vi "SaveVI.vi"(0 "VI in":refnum<vi>, 5 "Project Path":path, 7 "Folder name":string, 9 "VI name":string, 11 "error in (no error)":errorcluster) -> (4 "VI out":refnum<vi>, 15 "error out":errorcluster)   [LabVIEW 2016, in "ScriptSubVIs.lvlib"]
doc: "Creates and saves the New VI in a given name"
uses:
  ScriptSubVIs.lvlib
  <vilib>/SLL Toolkit/SLL File IO/SLL File IO.lvlib
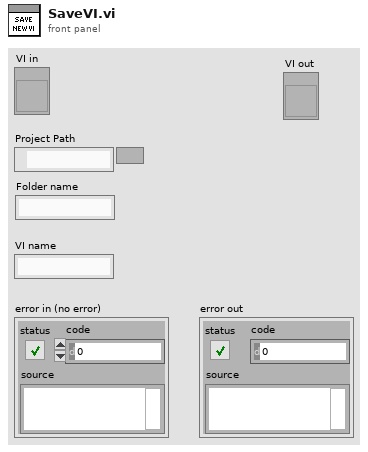
[diagram p1: front panel]
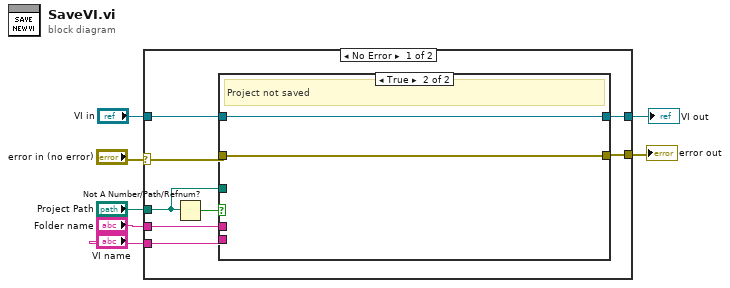
[diagram p0: block diagram]
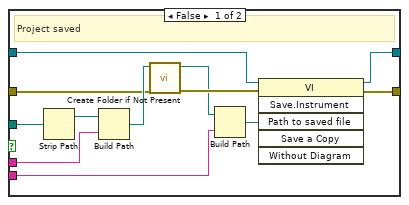
[diagram p2: hidden frame]
diagram:
  n1 = case shown="No Error" "error in (no error)" {
    selector: "error in (no error)" -> [w14 w30]
    tunnel: [w15 w30] -> w7
    tunnel: "VI name" -> [w13 _]
    tunnel: "VI in" -> [w12 w31]
    tunnel: "Project Path" -> [w11 _]
    tunnel: [w9 w31] -> w2
    tunnel: "Folder name" -> [w8 _]
    frame No Error {
      n2 = Not A Number/Path/Refnum?(number/path/refnum=w11) -> (NaN/Path/Refnum?=w10:bool)
      n3 = case shown="True" w10 {
        tunnel: w14 -> [w21 w29]
        tunnel: [w25 w29] -> w15
        tunnel: w12 -> [w27 w28]
        tunnel: [w26 w28] -> w9
        tunnel: w11 -> [w24 _]
        tunnel: w13 -> [w18 _]
        tunnel: w8 -> [w16 _]
        frame False {
          # "Project saved"
          n4 = Strip Path(path=w24) -> (stripped path=w23:path)  [unwired: 1 out]
          n5 = Build Path(base path=w23, name or relative path=w16) -> (appended path=w22:path)
          n6 = call <vilib>:"Create Folder if Not Present.vi"("error in (no error)"=w21, "Path"=w22) -> ("error out"=w20:errorcluster, "Path out"=w19:path)  [unwired: 8 in]
          n7 = Build Path(base path=w19, name or relative path=w18) -> (appended path=w17:path)
          n8 = invoke class="VI" method="Save.Instrument"(reference=w27, error in=w20, "Path to saved file"=w17) -> (reference out=w26:refnum<vi>, error out=w25:errorcluster)  [unwired: 3 in, 4 out]
        }
        frame True {
          # "Project not saved"
        }
      }
    }
    frame Error {
    }
  }
  "error out" <- w7
  "VI out" <- w2
